vi "条件结构的使用(下).vi"() -> ()   [LabVIEW 2018]
panel:
  out "状态指示":bool
  out "当前状态栏":string
  in  "当前温度":dbl
  in  "最高温度":dbl
  in  "最小液位":dbl
  in  "当前液位":dbl
  in  "最大液位":dbl
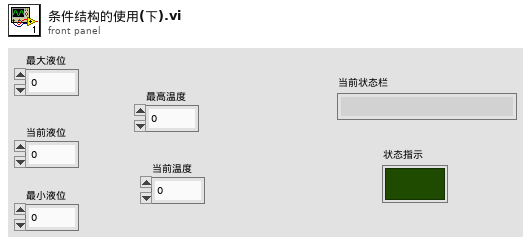
[diagram p1: front panel]
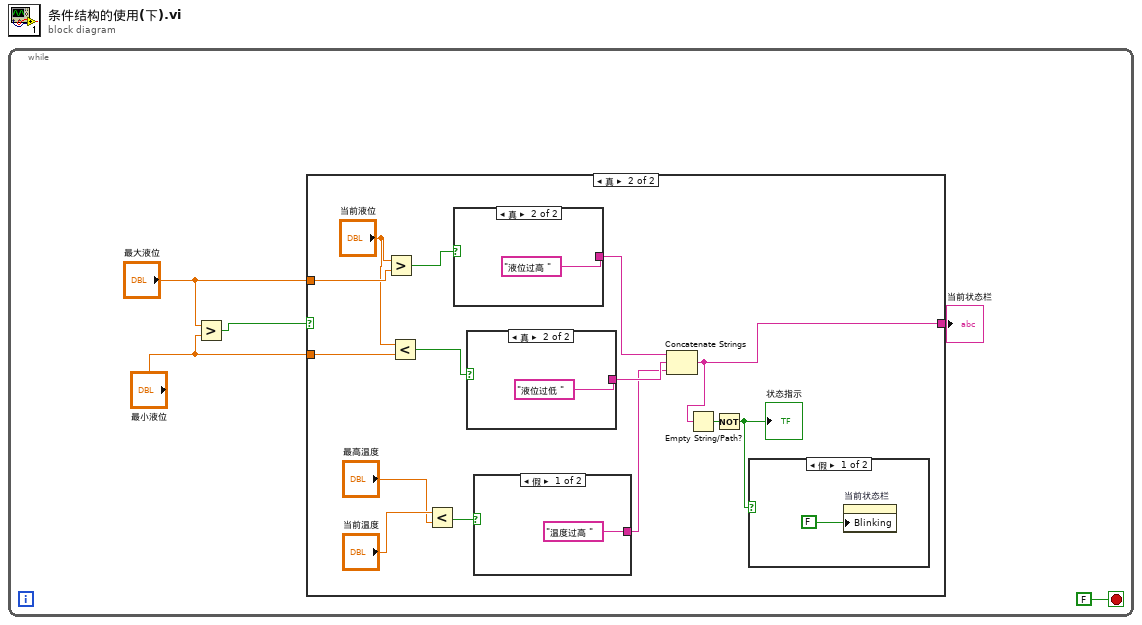
[diagram p0: block diagram]
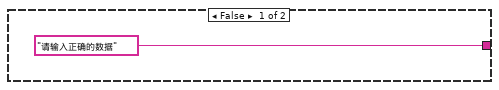
[diagram p2: hidden frame]
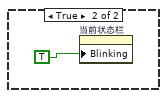
[diagram p3: hidden frame]
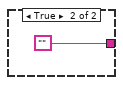
[diagram p4: hidden frame]
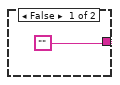
[diagram p5: hidden frame]
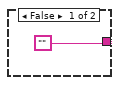
[diagram p6: hidden frame]
diagram:
  n1 = while {
    stop <- FALSE stop-if-true
    n2 = Greater?(x="最大液位", y="最小液位") -> (0:w4:bool)
    n3 = case shown="真" w4 {
      tunnel: ["请输入正确的数据" w9] -> w3
      tunnel: "最大液位" -> [_ w20]
      tunnel: "最小液位" -> [_ w17]
      frame False {
      }
      frame True {
        n4 = Greater?(x="当前液位", y=w20) -> (0:w19:bool)
        n5 = Less?(x="当前液位", y=w17) -> (x < y?=w16:bool)
        n6 = Less?(x="当前温度", y="最高温度") -> (x < y?=w13:bool)
        n7 = case shown="真" w19 {
          tunnel: ["" "液位过高 "] -> w12
          frame False {
          }
          frame True {
          }
        }
        n8 = case shown="真" w16 {
          tunnel: ["" "液位过低 "] -> w11
          frame False {
          }
          frame True {
          }
        }
        n9 = case shown="假" w13 {
          tunnel: ["温度过高 " ""] -> w10
          frame False {
          }
          frame True {
          }
        }
        n10 = Concatenate Strings(w12, w11, w10) -> (w9:string)
        n11 = Empty String/Path?(string/path=w9) -> (empty?=w8:bool)
        n12 = Not(x=w8) -> (.not. x?=w7:bool)
        "状态指示" <- w7
        n13 = case shown="假" w7 {
          frame False {
            n14 = property on="当前状态栏" class="Str"("Blinking"=FALSE) -> ()  [unwired: 2 in, 2 out]
          }
          frame True {
            n15 = property on="当前状态栏" class="Str"("Blinking"=TRUE) -> ()  [unwired: 2 in, 2 out]
          }
        }
      }
    }
    "当前状态栏" <- w3
  }
